vi "CreateImage.vi"() -> ()   [LabVIEW 2020]
panel:
  in  "NumImages":i32
  in  "CreateNegImages":bool
  in  "CreatePosImages":bool
  in  "ExportNeg":bool
  in  "Triangle":bool
  in  "NumOvals":i32
  in  "NumRectangles":i32
  in  "stop":bool
  in  "ExportPos":bool
  in  "CreateImage":bool
  out "height":dbl
  out "y":dbl
  out "width":dbl
  out "x":dbl
  out "2D Picture":picture
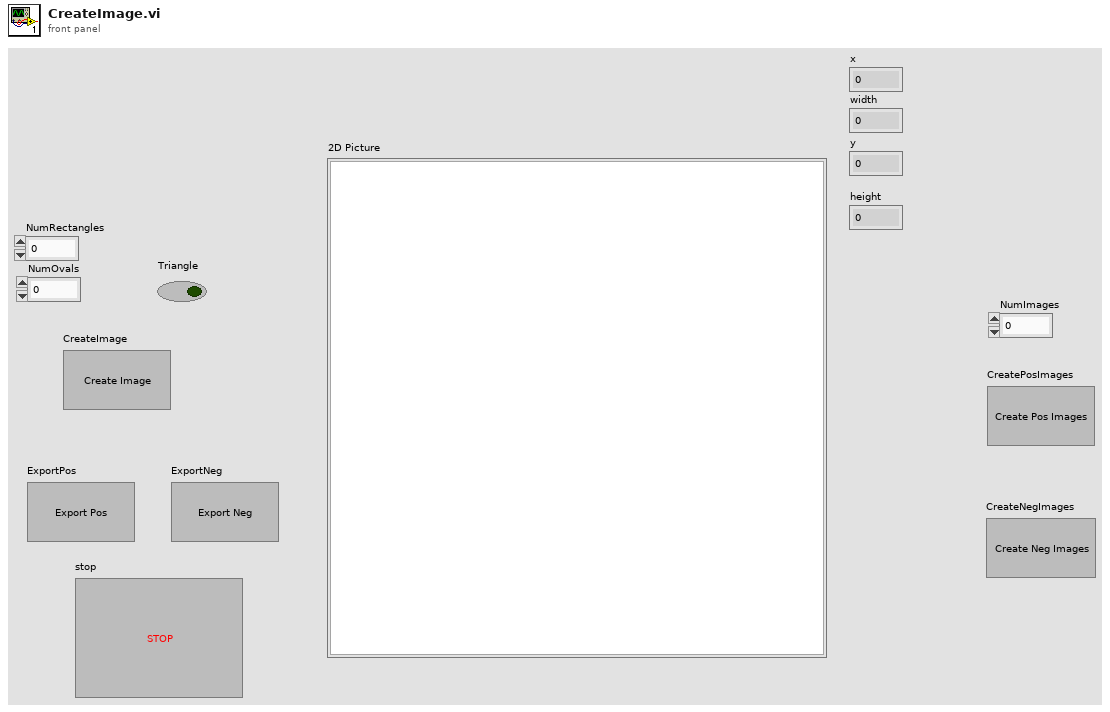
[diagram p1: front panel]
types:
  T1 = cluster{"left":i16, "top":i16, "right":i16, "bottom":i16}
  T2 = enum16{"open", "replace", "create", "open or create", "replace or create", "replace or create with confirmation"}
  T3 = cluster{"Width":u16, "Style":enum32{"Solid", "Dash", "Dot", "DashDot", "DashDotDot"}}
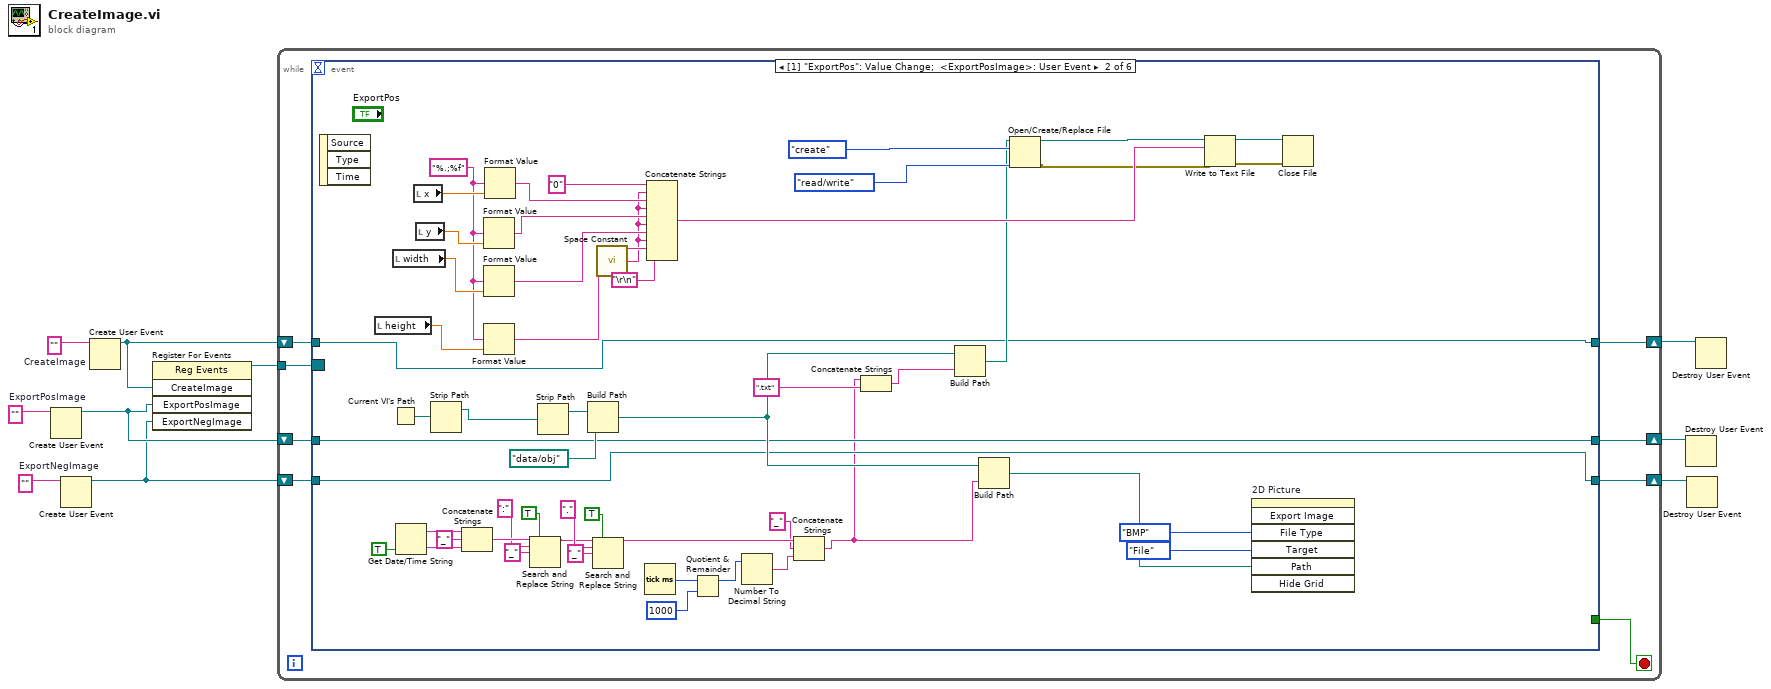
[diagram p0: block diagram]
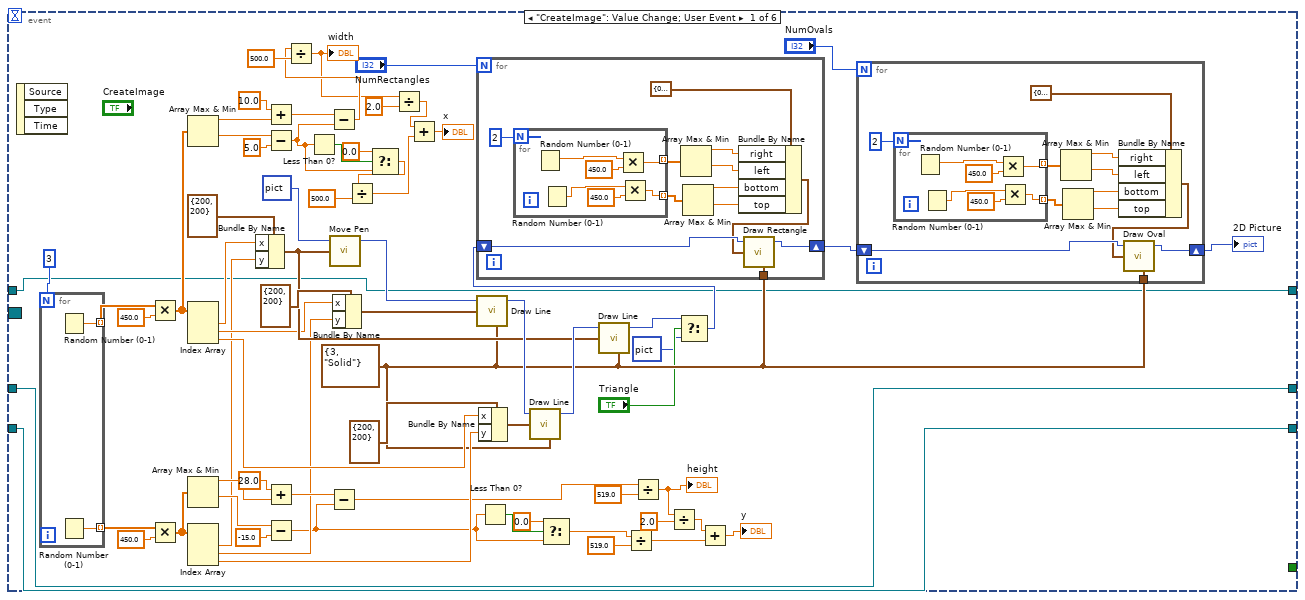
[diagram p2: hidden frame]
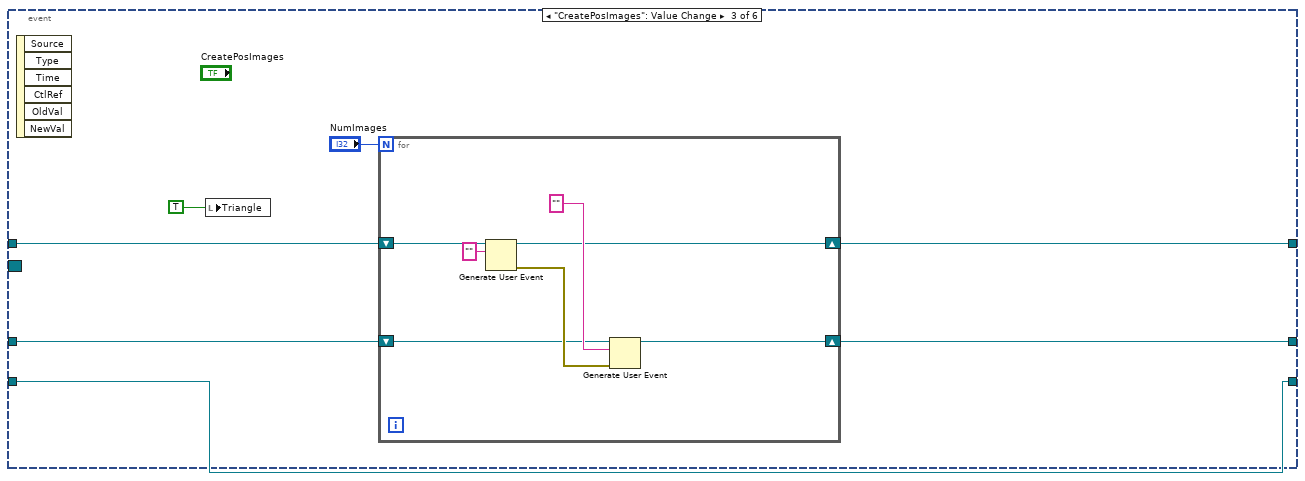
[diagram p3: hidden frame]
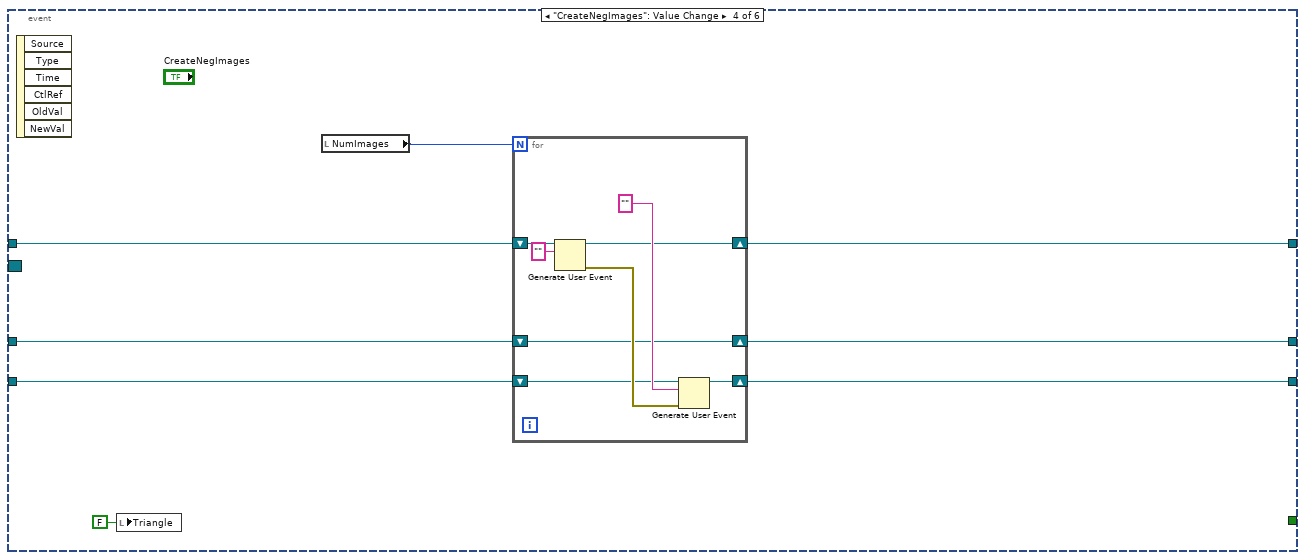
[diagram p4: hidden frame]
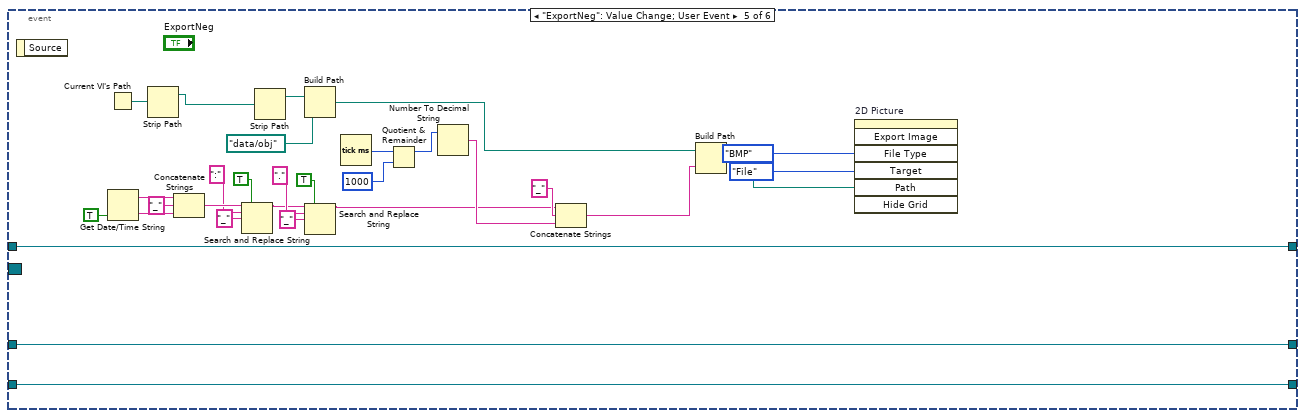
[diagram p5: hidden frame]
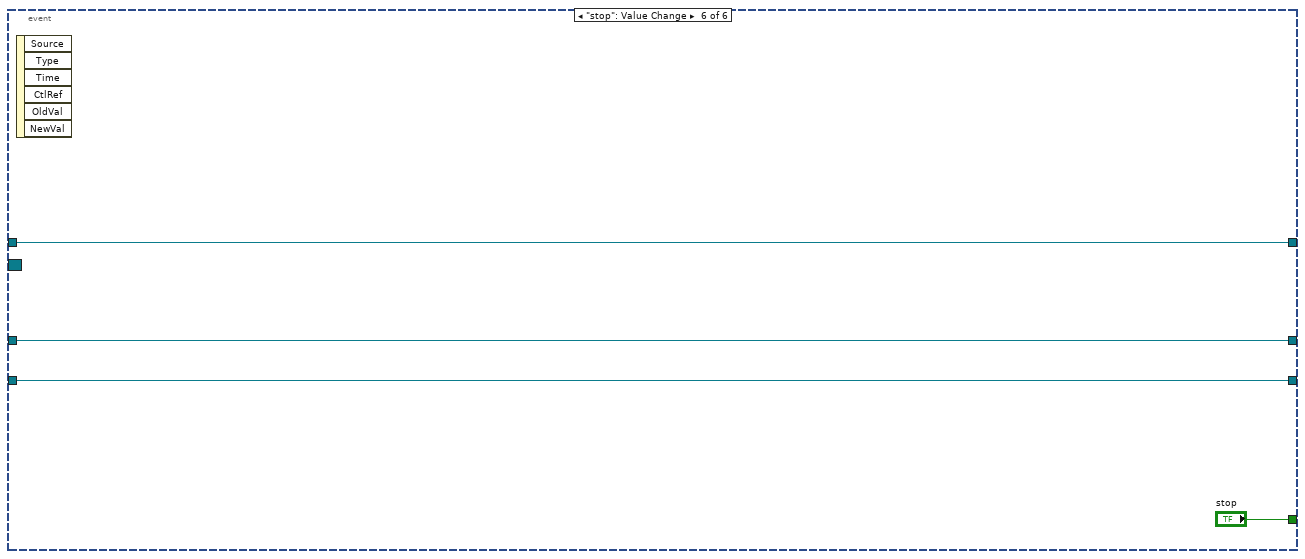
[diagram p6: hidden frame]
diagram:
  w4 = ""  # ExportNegImage
  w6 = ""  # ExportPosImage
  w10 = ""  # CreateImage
  n1 = Create User Event(user event datatype=w6) -> (user event=w5:refnum<user-event>)  [unwired: 1 in, 1 out]
  n2 = Create User Event(user event datatype=w4) -> (user event=w3:refnum<user-event>)  [unwired: 1 in, 1 out]
  n3 = Create User Event(user event datatype=w10) -> (user event=w8:refnum<user-event>)  [unwired: 1 in, 1 out]
  n4 = register-events(w8, w5, w3) -> (reference out=w9:refnum<event-registration>)  [unwired: 2 in, 1 out]
  n5 = while {
    tunnel: w9 -> [w17]
    shift-right: [w15] -> w7
    shift-left: w8 -> [w16]
    shift-right: [w13] -> w2
    shift-left: w5 -> [w14]
    shift-right: [w11] -> w1
    shift-left: w3 -> [w12]
    stop <- w18 stop-if-true
    n6 = event shown="[1] \"ExportPos\": Value Change;  <ExportPosImage>: User Event" {
      selector: w17 -> [_ _ _ _ _ _]
      dyn-events: _ -> [_ _ _ _ _ _]
      timeout: _ -> [_ _ _ _ _ _]
      tunnel: [_ _ _ _ _ "stop"] -> w18
      tunnel: w16 -> [w29 w133 w184 w199 w217 w240]
      tunnel: [w29 w133 w183 w198 w217 w240] -> w15
      tunnel: w14 -> [w30 w134 w181 w196 w216 w239]
      tunnel: [w30 w134 w182 w197 w216 w239] -> w13
      tunnel: w12 -> [w31 w135 w179 w195 w215 w238]
      tunnel: [w31 w135 w179 w194 w215 w238] -> w11
      event "CreateImage": Value Change; User Event {
        w52 = T3 {"Width"=3, "Style"=enum."Solid"} ("pen")
        n7 = event-data() -> ()  [unwired: 1 in, 3 out]
        n8 = for {
          N: 3 -> [_]
          tunnel: [w125] -> w76 mode=indexing
          tunnel: [w124] -> w73 mode=indexing
          n9 = Random Number (0-1)() -> (number: 0 to 1=w125:dbl)
          n10 = Random Number (0-1)() -> (number: 0 to 1=w124:dbl)
        }
        n11 = Multiply(x=w76, y=450.0) -> (x*y=w72:dbl[])
        n12 = Multiply(x=w73, y=450.0) -> (x*y=w62:dbl[])
        n13 = Array Max & Min(array=w72) -> (max value=w69:dbl, min value=w71:dbl)  [unwired: 2 out]
        n14 = Index Array(array=w72) -> (element #1=w60:dbl, element #2=w59:dbl, element #3=w58:dbl)  [unwired: 3 in]
        n15 = Array Max & Min(array=w62) -> (max value=w64:dbl, min value=w63:dbl)  [unwired: 2 out]
        n16 = Index Array(array=w62) -> (element #1=w57:dbl, element #2=w56:dbl, element #3=w55:dbl)  [unwired: 3 in]
        n17 = Bundle By Name(cluster=cluster{"x":i16, "y":i16} {"x"=200, "y"=200} ("new position"), "x"=w60, "y"=w57) -> (w78:cluster{"x":i16, "y":i16})
        n18 = Add(x=10.0, y=w69) -> (x+y=w67:dbl)
        n19 = Subtract(x=w71, y=5.0) -> (x-y=w33:dbl)
        n20 = Add(x=28.0, y=w64) -> (x+y=w66:dbl)
        n21 = Subtract(x=w63, y=-15.0) -> (x-y=w38:dbl)
        n22 = Less Than 0?(x=w33) -> (x < 0?=w35:bool)
        n23 = Subtract(x=w67, y=w33) -> (x-y=w41:dbl)
        n24 = Divide(x=w41, y=500.0) -> (x/y=w23:dbl)
        "width" <- w23
        n25 = Subtract(x=w66, y=w38) -> (x-y=w45:dbl)
        n26 = call <vilib>:"Move Pen.vi"("new position"=w78, "picture"=picture data[5B]) -> ("new picture"=w86:picture)  [unwired: 3 in]
        n27 = Bundle By Name(cluster=cluster{"x":i16, "y":i16} {"x"=200, "y"=200} ("new position"), "x"=w59, "y"=w56) -> (w82:cluster{"x":i16, "y":i16})
        n28 = Select(t=0.0, s=w35, f=w33) -> (s? t:f=w32:dbl)
        n29 = Divide(x=w32, y=500.0) -> (x/y=w20:dbl)
        n30 = Divide(x=w23, y=2.0) -> (x/y=w19:dbl)
        n31 = Add(x=w19, y=w20) -> (x+y=→"x":dbl)
        n32 = call <vilib>:"Draw Line.vi"("picture"=w86, "end point"=w82, "pen"=w52) -> ("new picture"=w84:picture)  [unwired: 6 in]
        n33 = Bundle By Name(cluster=cluster{"x":i16, "y":i16} {"x"=200, "y"=200} ("new position"), "x"=w58, "y"=w55) -> (w81:cluster{"x":i16, "y":i16})
        n34 = Less Than 0?(x=w38) -> (x < 0?=w39:bool)
        n35 = call <vilib>:"Draw Line.vi"("picture"=w84, "end point"=w81, "pen"=w52) -> ("new picture"=w79:picture)  [unwired: 6 in]
        n36 = Select(t=0.0, s=w39, f=w38) -> (s? t:f=w36:dbl)
        n37 = call <vilib>:"Draw Line.vi"("picture"=w79, "end point"=w78, "pen"=w52) -> ("new picture"=w48:picture)  [unwired: 6 in]
        n38 = Divide(x=w36, y=519.0) -> (x/y=w28:dbl)
        n39 = Divide(x=w45, y=519.0) -> (x/y=w27:dbl)
        "height" <- w27
        n40 = Divide(x=w27, y=2.0) -> (x/y=w25:dbl)
        n41 = Select(t=w48, s="Triangle", f=picture data[5B] ("picture")) -> (s? t:f=w47:picture)
        n42 = for {
          N: "NumRectangles" -> [_]
          shift-right: [w108] -> w53
          shift-left: w47 -> [w109]
          tunnel: w52 -> [w106]
          n43 = for {
            N: 2 -> [_]
            tunnel: [w121] -> w115 mode=indexing
            tunnel: [w120] -> w114 mode=indexing
            n44 = Random Number (0-1)() -> (number: 0 to 1=w119:dbl)
            n45 = Random Number (0-1)() -> (number: 0 to 1=w118:dbl)
            n46 = Multiply(x=w119, y=450.0) -> (x*y=w121:dbl)
            n47 = Multiply(x=w118, y=450.0) -> (x*y=w120:dbl)
          }
          n48 = Array Max & Min(array=w115) -> (max value=w113:dbl, min value=w112:dbl)  [unwired: 2 out]
          n49 = Array Max & Min(array=w114) -> (max value=w111:dbl, min value=w110:dbl)  [unwired: 2 out]
          n50 = Bundle By Name(cluster=T1 {"left"=0, "top"=0, "right"=0, "bottom"=0} ("rect"), "right"=w113, "left"=w112, "bottom"=w111, "top"=w110) -> (w107:T1)
          n51 = call <vilib>:"Draw Rectangle.vi"("picture"=w109, "rect"=w107, "pen"=w106) -> ("new picture"=w108:picture)  [unwired: 6 in]
        }
        n52 = Add(x=w25, y=w28) -> (x+y=→"y":dbl)
        n53 = for {
          N: "NumOvals" -> [_]
          shift-right: [w90] -> w50
          shift-left: w53 -> [w91]
          tunnel: w52 -> [w88]
          n54 = for {
            N: 2 -> [_]
            tunnel: [w103] -> w97 mode=indexing
            tunnel: [w102] -> w96 mode=indexing
            n55 = Random Number (0-1)() -> (number: 0 to 1=w101:dbl)
            n56 = Random Number (0-1)() -> (number: 0 to 1=w100:dbl)
            n57 = Multiply(x=w101, y=450.0) -> (x*y=w103:dbl)
            n58 = Multiply(x=w100, y=450.0) -> (x*y=w102:dbl)
          }
          n59 = Array Max & Min(array=w97) -> (max value=w95:dbl, min value=w94:dbl)  [unwired: 2 out]
          n60 = Array Max & Min(array=w96) -> (max value=w93:dbl, min value=w92:dbl)  [unwired: 2 out]
          n61 = Bundle By Name(cluster=T1 {"left"=0, "top"=0, "right"=0, "bottom"=0} ("rect"), "right"=w95, "left"=w94, "bottom"=w93, "top"=w92) -> (w89:T1)
          n62 = call <vilib>:"Draw Oval.vi"("picture"=w91, "rect"=w89, "pen"=w88) -> ("new picture"=w90:picture)  [unwired: 6 in]
        }
        "2D Picture" <- w50
      }
      event "ExportPos": Value Change; User Event {
        w136 = "%.;%f" ("format string")
        n63 = event-data() -> ()  [unwired: 1 in, 3 out]
        n64 = local read "height"() -> (w139:dbl)
        n65 = Current VI's Path() -> (path=w154:path)
        n66 = local read "width"() -> (w138:dbl)
        n67 = Get Date/Time String(want seconds? (F)=TRUE) -> (date string=w175:string, time string=w174:string)  [unwired: 2 in]
        n68 = local read "x"() -> (w140:dbl)
        n69 = local read "y"() -> (w137:dbl)
        n70 = Strip Path(path=w154) -> (stripped path=w141:path)  [unwired: 1 out]
        n71 = Concatenate Strings(w175, "_" ("string"), w174) -> (w167:string)
        n72 = Format Value(format string=w136, value (0)=w137) -> (output string=w170:string)  [unwired: 1 in]
        n73 = Format Value(format string=w136, value (0)=w138) -> (output string=w169:string)  [unwired: 1 in]
        n74 = Format Value(format string=w136, value (0)=w139) -> (output string=w168:string)  [unwired: 1 in]
        n75 = Format Value(format string=w136, value (0)=w140) -> (output string=w171:string)  [unwired: 1 in]
        n76 = Search and Replace String(replace all?=TRUE ("replace all? (F)"), input string=w167, search string=":", replace string="_" ("replace string (\"\")")) -> (result string=w160:string)  [unwired: 4 in, 3 out]
        n77 = Strip Path(path=w141) -> (stripped path=w149:path)  [unwired: 1 out]
        n78 = Build Path(base path=w149, name or relative path=path "data/obj") -> (appended path=w147:path)
        n79 = Search and Replace String(replace all?=TRUE ("replace all? (F)"), input string=w160, search string=".", replace string="_" ("replace string (\"\")")) -> (result string=w130:string)  [unwired: 4 in, 3 out]
        n80 = call <vilib>:"Space Constant.vi"() -> ("String"=w151:string)
        n81 = Tick Count (ms)() -> (millisecond timer value=w132:u32)
        n82 = Concatenate Strings("0" ("string"), w151, w171, w151, w170, w151, w169, w151, w168, "\r\n") -> (w153:string)
        n83 = Quotient & Remainder(x=w132, y=u32 1000) -> (x-y*floor(x/y)=w127:u32)  [unwired: 1 out]
        n84 = Number To Decimal String(number=w127) -> (decimal integer string=w128:string)  [unwired: 1 in]
        n85 = Concatenate Strings(w130, "_" ("string"), w128) -> (w126:string)
        n86 = Concatenate Strings(w126, ".txt" ("string")) -> (w145:string)
        n87 = Build Path(base path=w147, name or relative path=w145) -> (appended path=w144:path)
        n88 = Build Path(base path=w147, name or relative path=w126) -> (appended path=w172:path)
        n89 = Open/Create/Replace File(file path (use dialog)=w144, operation (0:open)=T2."create", access (0:read/write)=enum16{"read/write", "read-only", "write-only"}."read/write") -> (refnum out=w143:refnum<file>, error out=w142:errorcluster)  [unwired: 3 in, 1 out]
        n90 = Write to Text File(file (use dialog)=w143, text=w153, error in=w142) -> (refnum out=w158:refnum<file>, error out=w157:errorcluster)  [unwired: 1 in, 1 out]
        n91 = invoke on="2D Picture" class="Pict" method="Export Image"("File Type"=enum32{"BMP", "EPS", "EMF", "PICT"}."BMP", "Target"=enum32{"File", "Clipboard"}."File", "Path"=w172) -> ()  [unwired: 4 in, 7 out]
        n92 = Close File(refnum=w158, error in=w157) -> ()  [unwired: 2 out]
      }
      event "CreatePosImages": Value Change {
        n93 = event-data() -> ()  [unwired: 1 in, 6 out]
        n94 = local write "Triangle"(TRUE) -> ()
        n95 = for {
          N: "NumImages" -> [_]
          shift-right: [w186] -> w183
          shift-left: w184 -> [w191]
          shift-right: [w185] -> w182
          shift-left: w181 -> [w187]
          n96 = Generate User Event(user event=w191, event data cluster="" ("event data")) -> (user event out=w186:refnum<user-event>, error out=w188:errorcluster)  [unwired: 2 in]
          n97 = Generate User Event(user event=w187, event data cluster="" ("event data"), error in=w188) -> (user event out=w185:refnum<user-event>)  [unwired: 1 in, 1 out]
        }
      }
      event "CreateNegImages": Value Change {
        n98 = event-data() -> ()  [unwired: 1 in, 6 out]
        n99 = local write "Triangle"(FALSE ("Triangle")) -> ()
        n100 = local read "NumImages"() -> (w192:i32)
        n101 = for {
          N: w192 -> [_]
          shift-right: [w203] -> w198
          shift-left: w199 -> [w207]
          shift-right: [w201] -> w197
          shift-left: w196 -> [w201]
          shift-right: [w200] -> w194
          shift-left: w195 -> [w202]
          n102 = Generate User Event(user event=w207, event data cluster="" ("event data")) -> (user event out=w203:refnum<user-event>, error out=w204:errorcluster)  [unwired: 2 in]
          n103 = Generate User Event(user event=w202, event data cluster="" ("event data"), error in=w204) -> (user event out=w200:refnum<user-event>)  [unwired: 1 in, 1 out]
        }
      }
      event "ExportNeg": Value Change; User Event {
        n104 = event-data() -> ()  [unwired: 1 in, 1 out]
        n105 = Current VI's Path() -> (path=w223:path)
        n106 = Get Date/Time String(want seconds? (F)=TRUE) -> (date string=w235:string, time string=w234:string)  [unwired: 2 in]
        n107 = Strip Path(path=w223) -> (stripped path=w219:path)  [unwired: 1 out]
        n108 = Concatenate Strings(w235, "_" ("string"), w234) -> (w232:string)
        n109 = Search and Replace String(replace all?=TRUE ("replace all? (F)"), input string=w232, search string=":", replace string="_" ("replace string (\"\")")) -> (result string=w225:string)  [unwired: 4 in, 3 out]
        n110 = Strip Path(path=w219) -> (stripped path=w222:path)  [unwired: 1 out]
        n111 = Build Path(base path=w222, name or relative path=path "data/obj") -> (appended path=w220:path)
        n112 = Search and Replace String(replace all?=TRUE ("replace all? (F)"), input string=w225, search string=".", replace string="_" ("replace string (\"\")")) -> (result string=w209:string)  [unwired: 4 in, 3 out]
        n113 = Tick Count (ms)() -> (millisecond timer value=w214:u32)
        n114 = Quotient & Remainder(x=w214, y=u32 1000) -> (x-y*floor(x/y)=w210:u32)  [unwired: 1 out]
        n115 = Number To Decimal String(number=w210) -> (decimal integer string=w211:string)  [unwired: 1 in]
        n116 = Concatenate Strings(w209, "_" ("string"), w211) -> (w208:string)
        n117 = Build Path(base path=w220, name or relative path=w208) -> (appended path=w218:path)
        n118 = invoke on="2D Picture" class="Pict" method="Export Image"("File Type"=enum32{"BMP", "EPS", "EMF", "PICT"}."BMP", "Target"=enum32{"File", "Clipboard"}."File", "Path"=w218) -> ()  [unwired: 4 in, 7 out]
      }
      event "stop": Value Change {
        n119 = event-data() -> ()  [unwired: 1 in, 6 out]
      }
    }
  }
  n120 = Destroy User Event(user event=w2) -> ()  [unwired: 1 in, 1 out]
  n121 = Destroy User Event(user event=w1) -> ()  [unwired: 1 in, 1 out]
  n122 = Destroy User Event(user event=w7) -> ()  [unwired: 1 in, 1 out]
